vi "Write Acquisition Status.vi"(0 "acquisition in progress":bool, 2 "shared":refnum<class "niUSRP Rx Core v1 FPGA.lvclass">=refnum, 5 "waiting for trigger":bool) -> ()   [LabVIEW 2023]
doc: "this VI is used to transfer acquisition statuses across clock domains; from the Acquisition Loop to the ActiveLED configuration."
uses:
  <vilib>/rvi/DataTransferAndStorage/Container/XNode/niFpgaContainer.xnode
  <vilib>/rvi/DataTransferAndStorage/Register/Emulation/niFpgaRegisterEmulationRefIn.vi
  <instrlib>/niVST/Reference FPGA/FPGA/niUSRP Rx Core v1 FPGA/niUSRP Rx Core v1 FPGA.lvclass
  <instrlib>/niUSRP/Reference FPGA/Rx Core/niUSRP Rx Core v1 FPGA.lvclass
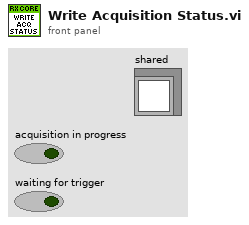
[diagram p1: front panel]
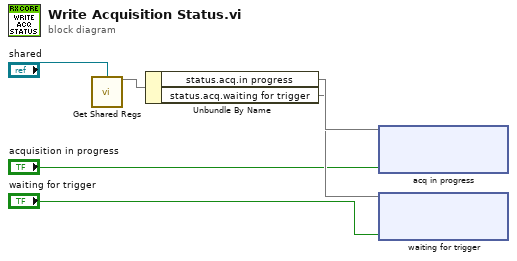
[diagram p0: block diagram]
diagram:
  n1 = call-dynamic "Get Shared Regs.vi"("shared"="shared") -> (4:w5)  [unwired: 14 in]
  n2 = Unbundle By Name(w5) -> ("status.acq.in progress"=w4, "status.acq.waiting for trigger"=w3)
  n3 = xnode "acq in progress"("Data"="acquisition in progress", "Register In"=w4) -> ()  [unwired: 1 out]
  n4 = xnode "waiting for trigger"("Data"="waiting for trigger", "Register In"=w3) -> ()  [unwired: 1 out]
